vi "Sans titre 4.vi"() -> ()   [LabVIEW 2020]
uses:
  <vilib>/addons/database/Connection.llb/DB Tools Open Connec (String).vi
  <vilib>/addons/database/Connection.llb/Conn Execute.vi
  <vilib>/addons/database/Recordset.llb/Rec Fetch String Data (R).vi
  <vilib>/addons/database/Recordset.llb/Rec Destroy - Connection.vi
  <vilib>/addons/database/NI_Database_API.lvlib
panel:
  out "data":string
  out "error out":errorcluster
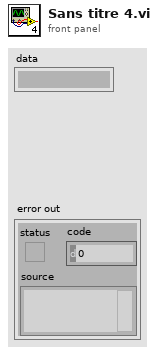
[diagram p1: front panel]
types:
  T1 = typedef "NI_Database_API.lvlib/Conn ObjectReference.ctl" = refnum<k1>
  T2 = typedef "NI_Database_API.lvlib/Rec ObjectReference.ctl" = refnum<k1>
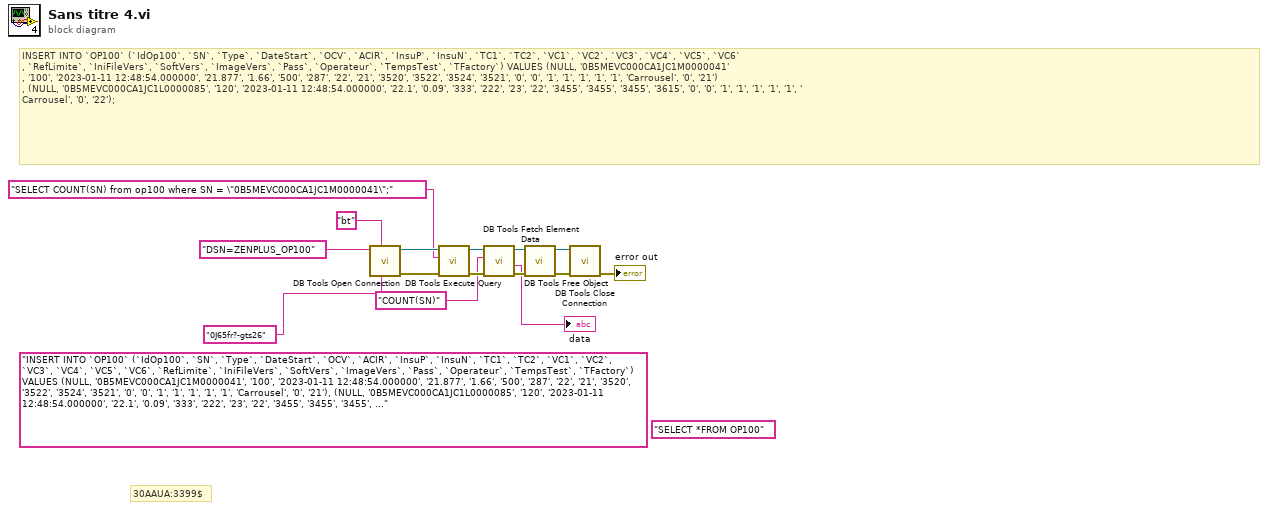
[diagram p0: block diagram]
diagram:
  (unwired) "SELECT *FROM OP100" ("SQL query")
  (unwired) "INSERT INTO `OP100` (`IdOp100`, `SN`, `Type`, `DateStart`, `OCV`, `ACIR`, `InsuP`, `InsuN`, `TC1`, `TC2`, `VC1`, `VC2`, `VC3`, `VC4`, `VC5`, `VC6`, `RefLimite`, `IniFileVers`, `SoftVers`, `ImageVers`, `Pass`, `Operateur`, `TempsTest`, `TFactory`) VALUES (NULL, '0B5MEVC000CA1JC1M0000041', '100', '2023-01-11 12:48:54.000000', '21.877', '1.66', '500', '287', '22', '21', '3520', '3522', '3524', '3521', '0', '0', '1', '1', '1', '1', '1', 'Carrousel', '0', '21'), (NULL, '0B5MEVC000CA1JC1L0000085', '120', '2023-01-11 12:48:54.000000', '22.1', '0.09', '333', '222', '23', '22', '3455', '3455', '3455', '3615', '0', '0', '1', '1', '1', '1', '1', 'Carrousel', '0', '22');" ("SQL query")
  # "30AAUA:3399$"
  # "INSERT INTO `OP100` (`IdOp100`, `SN`, `Type`, `DateStart`, `OCV`, `ACIR`, `InsuP`, `InsuN`, `TC1`, `TC2`, `VC1`, `VC2`, `VC3`, `VC4`, `VC5`, `VC6`\n, `RefLimite`, `IniFileVers`, `SoftVers`, `ImageVers`, `Pass`, `Operateur`, `TempsTest`, `TFactory`) VALUES (NULL, '0B5MEVC000CA1JC1M0000041'\n, '100', '2023-01-11 12:48:54.000000', '21.877', '1.66', '500', '287', '22', '21', '3520', '3522', '3524', '3521', '0', '0', '1', '1', '1', '1', '1', 'Carrousel', '0', '21')\n, (NULL, '0B5MEVC000CA1JC1L0000085', '120', '2023-01-11 12:48:54.000000', '22.1', '0.09', '333', '222', '23', '22', '3455', '3455', '3455', '3615', '0', '0', '1', '1', '1', '1', '1', '\nCarrousel', '0', '22');"
  n1 = call-poly <vilib>:"DB Tools Open Connection.vi"("password"="0J65fr?-gts26", "userID"="bt", "connection information"="DSN=ZENPLUS_OP100") -> ("error out"=w15:errorcluster, "connection reference"=w13:T1)  [unwired: 5 in]
  n2 = call-poly <vilib>:"DB Tools Execute Query.vi"("error in (no error)"=w15, "SQL query"="SELECT COUNT(SN) from op100 where SN = \"0B5MEVC000CA1JC1M0000041\";", "connection reference"=w13) -> ("error out"=w6:errorcluster, "recordset reference"=w5:T2)  [unwired: 5 in]
  n3 = call-poly <vilib>:"DB Tools Fetch Element Data.vi"("error in (no error)"=w6, "column index"="COUNT(SN)" ("type"), "recordset reference"=w5) -> ("error out"=w7:errorcluster, "data"=→"data":string, "recordset reference out"=w4:T2)  [unwired: 4 in]
  n4 = call-poly <vilib>:"DB Tools Free Object.vi"("error in (no error)"=w7, "recordset reference"=w4) -> ("error out"=w14:errorcluster, "connection reference"=w12:T1)  [unwired: 8 in]
  n5 = call <vilib>:"DB Tools Close Connection.vi"("error in (no error)"=w14, "connection reference"=w12) -> ("error out"=→"error out":errorcluster)  [unwired: 5 in]
